vi "Generate Waveform.vi"(8 "error in (no error)":errorcluster, 11 "Signal Generator in":refnum<class "Signal Generator.lvclass">) -> (0 "error out":errorcluster, 3 "Signal Generator out":refnum<class "Signal Generator.lvclass">)   [LabVIEW 2020, in "Signal Generator.lvlib" / "Signal Generator.lvclass"]
uses:
  Signal Generator.lvclass
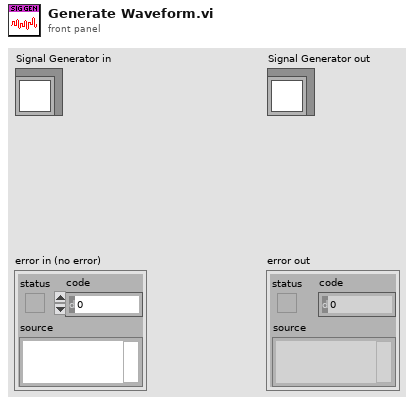
[diagram p1: front panel]
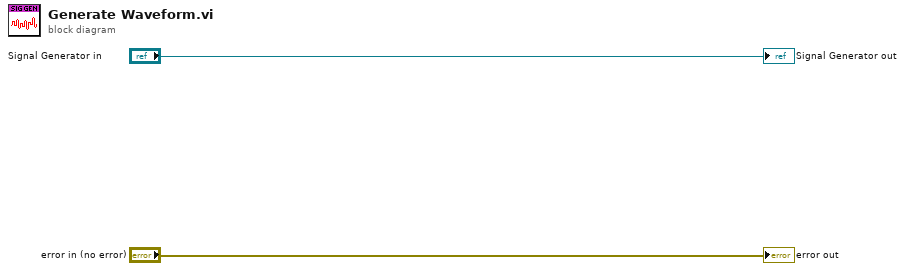
[diagram p0: block diagram]
diagram:
  "error out" <- "error in (no error)"
  "Signal Generator out" <- "Signal Generator in"
